vi "Apply.vi"(8 "error in":errorcluster, 11 "AI DAQmx Cont CFG Simulated in":refnum<class "AI DAQmx Cont CFG Simulated.lvclass">) -> (0 "error out":errorcluster, 3 "AI DAQmx Cont CFG Simulated out":refnum<class "AI DAQmx Cont CFG Simulated.lvclass">)   [LabVIEW 2023, in "DAQmx Simulated CFGs.lvlib" / "AI DAQmx Cont CFG Simulated.lvclass"]
uses:
  AI DAQmx Cont CFG Simulated.lvclass
  Configuration/Configuration JSON/Configuration JSON Base/CFG JSON.lvclass
  AI Current DAQmx Cont CFG/AI Current DAQmx Cont CFG.lvclass
  D:/git/HAL/HAL GOOP4/AI/AI Current DAQmx Cont CFG/AI Current DAQmx Cont CFG.lvclass
  D:/git/HAL/HAL GOOP4/DAQmx/DAQmx BufferLastReadsDBL/DAQmx BufferLastReadsDBL.lvclass
  D:/git/HAL/HAL GOOP4/DAQmx/DAQmx Base CFG/DAQmx Base CFG.lvclass
  D:/git/HAL/HAL GOOP4/CFG Target/CFG Target.lvclass
  D:/git/HAL/HAL GOOP4/Configuration/Configuration Semaphore/CFG Semaphore.lvclass
  D:/git/HAL/HAL GOOP4/Configuration/Configuration JSON/Configuration JSON Base/CFG JSON.lvclass
  D:/git/HAL/HAL GOOP4/Interfaces/IConfigure/IConfigure.lvclass
  D:/git/HAL/HAL GOOP4/AI/AI Simulated CFGs/AI DAQmx Cont CFG Simulated.lvclass
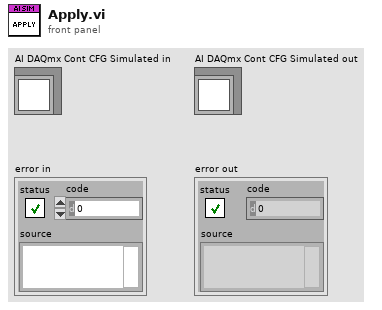
[diagram p1: front panel]
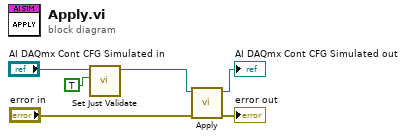
[diagram p0: block diagram]
diagram:
  n1 = call "Set Just Validate.vi"("Just Validate"=TRUE, "CFG JSON Base in"="AI DAQmx Cont CFG Simulated in") -> ("CFG JSON Base out"=w2:refnum<class "AI DAQmx Cont CFG Simulated.lvclass">)  [unwired: 9 in]
  n2 = call-parent "Apply.vi"("error in"="error in", "DAQmx Base CFG in"=w2) -> ("error out"=→"error out":errorcluster, "DAQmx Base CFG out"=→"AI DAQmx Cont CFG Simulated out":refnum<class "AI DAQmx Cont CFG Simulated.lvclass">)  [unwired: 8 in]
